vi "73XX Motion Controller Initialization VI.vi"(8 "error in (no error)":errorcluster, 10 "Custom XML":string, 11 "Device Item Ref in":T1 format="%.0x") -> (0 "error out":errorcluster, 3 "Device Item Ref out":T1 format="%.0x")   [LabVIEW 2010, in "73XX Motion Controller Custom Device.lvlib"]
uses:
  73XX Motion Controller Custom Device.lvlib
  <vilib>/NI VeriStand/Custom Device API/Custom Device Item Ref.ctl
  <vilib>/NI VeriStand/Custom Device API/Custom Device Channel.ctl
  <vilib>/NI VeriStand/Custom Device API/Custom Device Channel Type.ctl
  <vilib>/NI VeriStand/Custom Device API/Set Item Property (U16).vi
  <vilib>/NI Veristand/Custom Device API/Custom Device API.lvlib
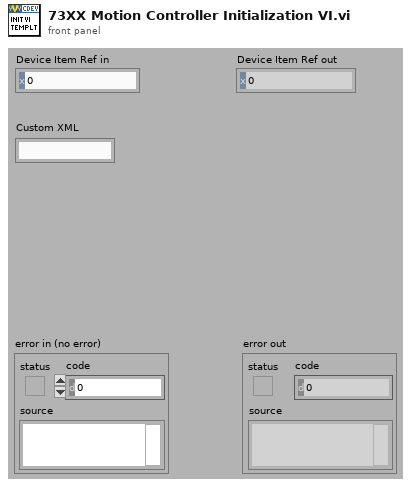
[diagram p1: front panel]
types:
  T1 = typedef "Custom Device API.lvlib/Custom Device Item Ref.ctl" = u64
  T2 = typedef "Custom Device API.lvlib/Custom Device Channel.ctl" = cluster{"Type":T3, "Units":string, "Default Value":dbl, "Faultable":bool, "Scalable":bool}
  T3 = typedef "Custom Device API.lvlib/Custom Device Channel Type.ctl" = enum16{"Input", "Output"}
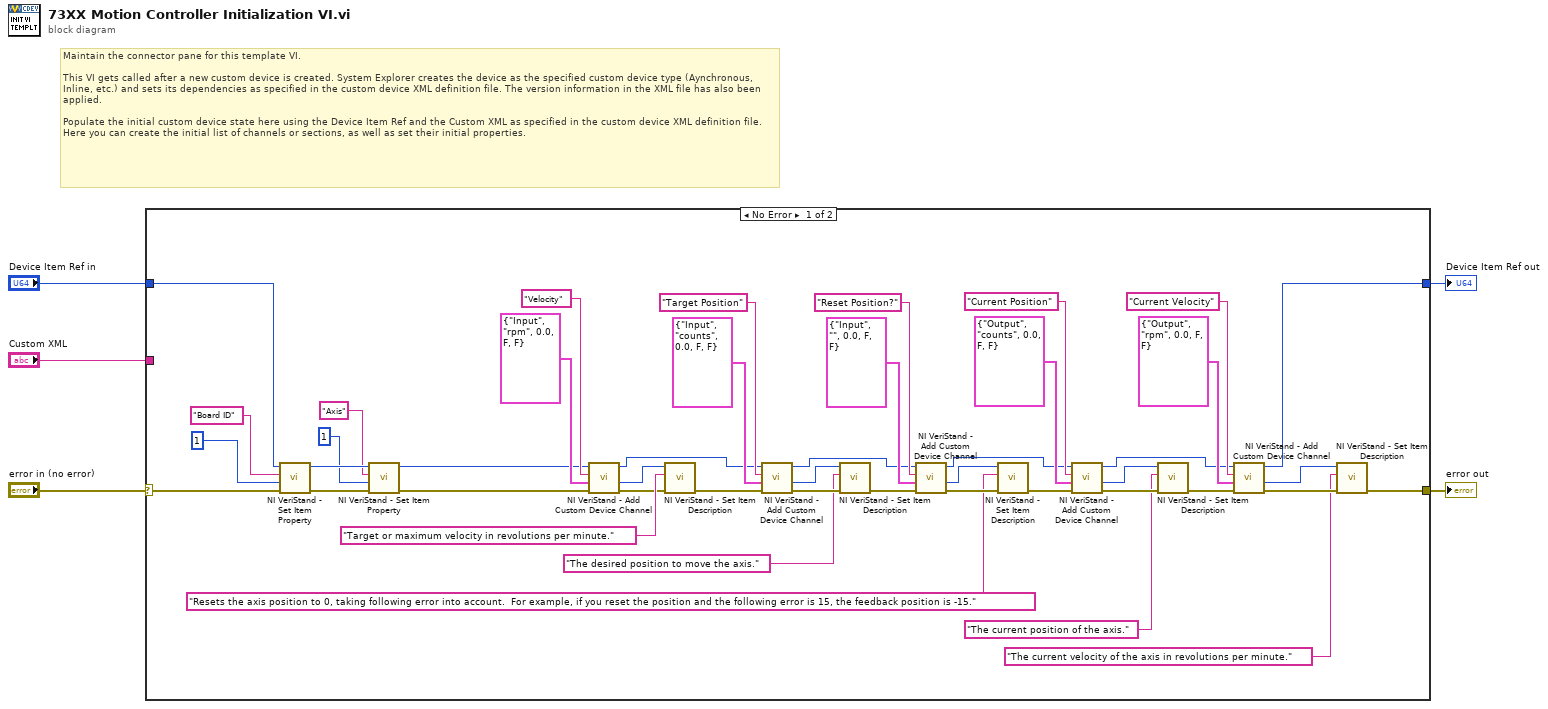
[diagram p0: block diagram]
diagram:
  # "Maintain the connector pane for this template VI.\n\nThis VI gets called after a new custom device is created. System Explorer creates the device as the specified custom device type (Aynchronous, Inline, etc.) and sets its dependencies as specified in the custom device XML definition file. The version information in the XML file has also been applied.\n\nPopulate the initial custom device state here using the Device Item Ref and the Custom XML as specified in the custom device XML definition file. Here you can create the initial list of channels or sections, as well as set their initial properties."
  n1 = case shown="No Error" "error in (no error)" {
    selector: "error in (no error)" -> [w45 w52]
    tunnel: [w25 w52] -> w5
    tunnel: [w34 w51] -> w3
    tunnel: "Device Item Ref in" -> [w50 w51]
    tunnel: "Custom XML" -> [_ _]
    frame No Error {
      n2 = call-poly <vilib>:"NI VeriStand - Set Item Property.vi"("error in (no error)"=w45, "Value"=u16 1, "Property Name"="Board ID", "Item Ref in"=w50) -> ("error out"=w39:errorcluster, "Item Ref out"=w40:T1)  [unwired: 5 in, 1 out]
      n3 = call-poly <vilib>:"NI VeriStand - Set Item Property.vi"("error in (no error)"=w39, "Value"=u16 1, "Property Name"="Axis", "Item Ref in"=w40) -> ("error out"=w42:errorcluster, "Item Ref out"=w41:T1)  [unwired: 5 in, 1 out]
      n4 = call <vilib>:"NI VeriStand - Add Custom Device Channel.vi"("error in (no error)"=w42, "Channel"=T2 {"Type"=enum."Input", "Units"="rpm", "Default Value"=0.0, "Faultable"=FALSE, "Scalable"=FALSE}, "Channel Name"="Velocity", "Parent Ref in"=w41) -> ("error out"=w27:errorcluster, "Channel Ref"=w29:T1, "Parent Ref out"=w14:T1)  [unwired: 4 in, 1 out]
      n5 = call <vilib>:"NI VeriStand - Set Item Description.vi"("error in (no error)"=w27, "Description"="Target or maximum velocity in revolutions per minute.", "Item Ref in"=w29) -> ("error out"=w15:errorcluster)  [unwired: 6 in, 2 out]
      n6 = call <vilib>:"NI VeriStand - Add Custom Device Channel.vi"("error in (no error)"=w15, "Channel"=T2 {"Type"=enum."Input", "Units"="counts", "Default Value"=0.0, "Faultable"=FALSE, "Scalable"=FALSE}, "Channel Name"="Target Position", "Parent Ref in"=w14) -> ("error out"=w17:errorcluster, "Channel Ref"=w12:T1, "Parent Ref out"=w13:T1)  [unwired: 4 in, 1 out]
      n7 = call <vilib>:"NI VeriStand - Set Item Description.vi"("error in (no error)"=w17, "Description"="The desired position to move the axis.", "Item Ref in"=w12) -> ("error out"=w16:errorcluster)  [unwired: 6 in, 2 out]
      n8 = call <vilib>:"NI VeriStand - Add Custom Device Channel.vi"("error in (no error)"=w16, "Channel"=T2 {"Type"=enum."Input", "Units"="", "Default Value"=0.0, "Faultable"=FALSE, "Scalable"=FALSE}, "Channel Name"="Reset Position?", "Parent Ref in"=w13) -> ("error out"=w19:errorcluster, "Channel Ref"=w11:T1, "Parent Ref out"=w10:T1)  [unwired: 4 in, 1 out]
      n9 = call <vilib>:"NI VeriStand - Set Item Description.vi"("error in (no error)"=w19, "Description"="Resets the axis position to 0, taking following error into account.  For example, if you reset the position and the following error is 15, the feedback position is -15.", "Item Ref in"=w11) -> ("error out"=w18:errorcluster)  [unwired: 6 in, 2 out]
      n10 = call <vilib>:"NI VeriStand - Add Custom Device Channel.vi"("error in (no error)"=w18, "Channel"=T2 {"Type"=enum."Output", "Units"="counts", "Default Value"=0.0, "Faultable"=FALSE, "Scalable"=FALSE}, "Channel Name"="Current Position", "Parent Ref in"=w10) -> ("error out"=w23:errorcluster, "Channel Ref"=w20:T1, "Parent Ref out"=w22:T1)  [unwired: 4 in, 1 out]
      n11 = call <vilib>:"NI VeriStand - Set Item Description.vi"("error in (no error)"=w23, "Description"="The current position of the axis.", "Item Ref in"=w20) -> ("error out"=w21:errorcluster)  [unwired: 6 in, 2 out]
      n12 = call <vilib>:"NI VeriStand - Add Custom Device Channel.vi"("error in (no error)"=w21, "Channel"=T2 {"Type"=enum."Output", "Units"="rpm", "Default Value"=0.0, "Faultable"=FALSE, "Scalable"=FALSE}, "Channel Name"="Current Velocity", "Parent Ref in"=w22) -> ("error out"=w26:errorcluster, "Channel Ref"=w24:T1, "Parent Ref out"=w34:T1)  [unwired: 4 in, 1 out]
      n13 = call <vilib>:"NI VeriStand - Set Item Description.vi"("error in (no error)"=w26, "Description"="The current velocity of the axis in revolutions per minute.", "Item Ref in"=w24) -> ("error out"=w25:errorcluster)  [unwired: 6 in, 2 out]
    }
    frame Error {
    }
  }
  "error out" <- w5
  "Device Item Ref out" <- w3
